vi "Init.vi"(8 "error in (no error)":errorcluster, 9 "Goal":T1, 10 "Start":T1, 11 "Adjacency":T2[][](array[typedef])) -> (0 "error out":errorcluster, 3 "Maze out":refnum<class "Maze.lvclass">)   [LabVIEW 2020, in "Maze.lvlib" / "Maze.lvclass"]
uses:
  Maze.lvclass
  Adjacency.ctl
  Position.ctl
  Maze.lvclass/Maze.ctl
  Maze.lvlib
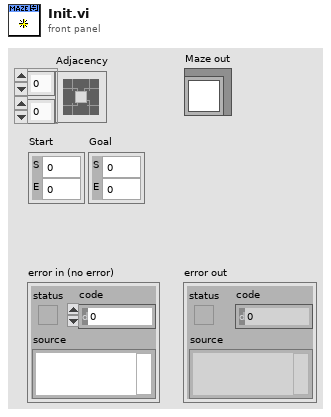
[diagram p1: front panel]
types:
  T1 = typedef "Maze.lvlib/Position.ctl" = cluster{"S":i32, "E":i32}
  T2 = typedef "Maze.lvlib/Adjacency.ctl" = cluster{"E":bool, "N":bool, "W":bool, "S":bool, "Goal":bool, "Start":bool}
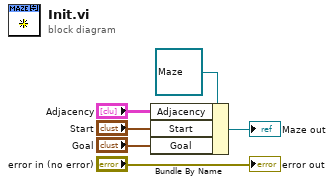
[diagram p0: block diagram]
diagram:
  n1 = Bundle By Name(cluster=refnum<class "Maze.lvclass"> refnum ("Maze in"), "Adjacency"="Adjacency", "Start"="Start", "Goal"="Goal") -> (→"Maze out":refnum<class "Maze.lvclass">)
  "error out" <- "error in (no error)"
